vi "Get Measurement Details.vi"(8 "error in":errorcluster) -> (0 "error out":errorcluster, 1 "measurement annotations":T1[](array[typedef]), 2 "service class":string, 3 "measurement details":T2)   [LabVIEW 2021, in "Keysight 34461A DMM Measurement.lvlib"]
uses:
  Keysight 34461A DMM Measurement.lvlib
  <vilib>/Plug-In SDKs/Measurements/NI Measurement Plug-In SDK.lvlib
  <vilib>/Plug-In SDKs/Measurements/Helpers/TypeDefs/Measurement Details.ctl
  <vilib>/Plug-In SDKs/Measurements/Helpers/TypeDefs/Measurement Annotation.ctl
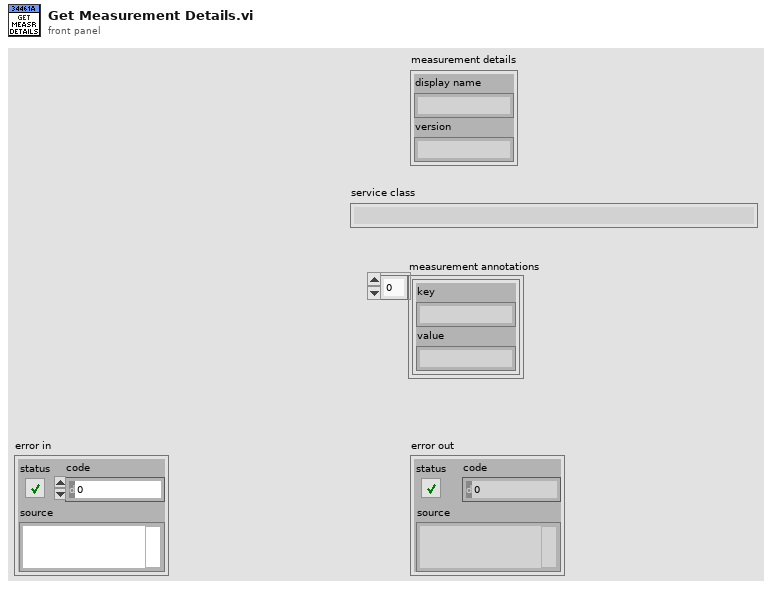
[diagram p1: front panel]
types:
  T1 = typedef "NI Measurement Plug-In SDK.lvlib/Measurement Annotation.ctl" = cluster{"key":string, "value":string}
  T2 = typedef "NI Measurement Plug-In SDK.lvlib/Measurement Details.ctl" = cluster{"display name":string, "version":string}
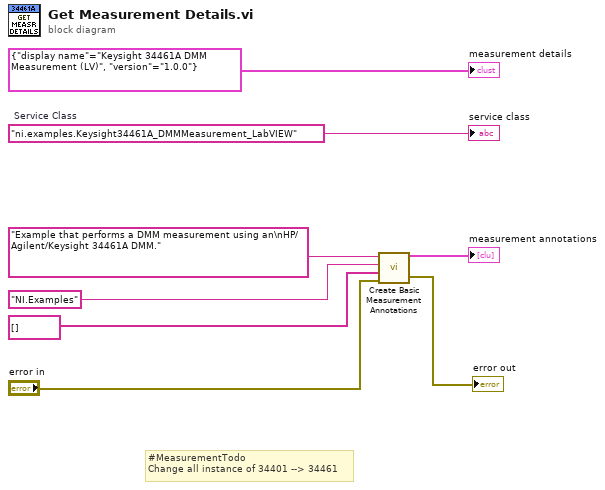
[diagram p0: block diagram]
diagram:
  w8 = "ni.examples.Keysight34461A_DMMMeasurement_LabVIEW"  # Service Class
  # "#MeasurementTodo\nChange all instance of 34401 --> 34461"
  n1 = call <vilib>:"Create Basic Measurement Annotations.vi"("error in"="error in", "tags"=string[] [] ("ni/service.tags"), "collection"="NI.Examples" ("ni/service.collection"), "description"="Example that performs a DMM measurement using an\nHP/Agilent/Keysight 34461A DMM." ("ni/service.description")) -> ("error out"=→"error out":errorcluster, "measurement annotations"=→"measurement annotations":T1[])  [unwired: 6 in]
  "measurement details" <- T2 {"display name"="Keysight 34461A DMM Measurement (LV)", "version"="1.0.0"} ("Measurement Details")
  "service class" <- w8
